vi "Periodic Tasks.vi"() -> ()   [LabVIEW 2019]
doc: "This VI runs in parallel to other tasks. It can contain as many user-defined periodic loops as you need. These can carry out PID or other sorts of timed response."
uses:
  <vilib>/Rock Robotics/WPI/DriverStation/WPI_DriverStationRobotMode2.ctl
  <vilib>/Rock Robotics/WPI/Solenoid/WPI_SolenoidValue.ctl
  <vilib>/Rock Robotics/WPI/Utilities/WPI_GetSetVariantRefNum.vi
  Robot Global Data.vi
  <vilib>/Rock Robotics/WPI/Solenoid/WPI_SolenoidSetEnum.vi
  <vilib>/Rock Robotics/Network Tables/NT Read Number.vi
  <vilib>/Rock Robotics/WPI/ThirdParty/Phoenix-LabVIEW/Motor Controller/Controls/CTRE_Phoenix_MotorControl_ControlMode.ctl
  <vilib>/Rock Robotics/WPI/ThirdParty/REV Robotics/SPARK MAX/Typedef/Spark MAX Control Type.ctl
  <vilib>/Rock Robotics/WPI/ThirdParty/Phoenix-LabVIEW/Motor Controller/Get/CTRE_Phoenix_MotorController_GetQuadratureData.vi
  <vilib>/Rock Robotics/WPI/ThirdParty/Phoenix-LabVIEW/Motor Controller/Get/CTRE_Phoenix_MotorController_GetSelectedSensorData.vi
  <vilib>/Rock Robotics/WPI/ThirdParty/Phoenix-LabVIEW/Motor Controller/Get/CTRE_Phoenix_MotorController_GetVoltage.vi
panel:
  out "Yaw":dbl
  out "status":dbl
  out "X position":dbl
  out "Y position":dbl
  in  "speed":dbl=1000.0
  in  "I Zone":dbl step=0.01
  in  "F Gain":dbl=2.1 step=0.01
  in  "D Gain":dbl=0.005 step=0.01
  in  "I Gain":dbl=0.019999999999999997 step=0.01
  in  "P Gain":dbl=4.0 min=0.0 step=0.01
  out "PID Chart":T1(graph)
  # "Click here to set max"
  # "Click here to set min"
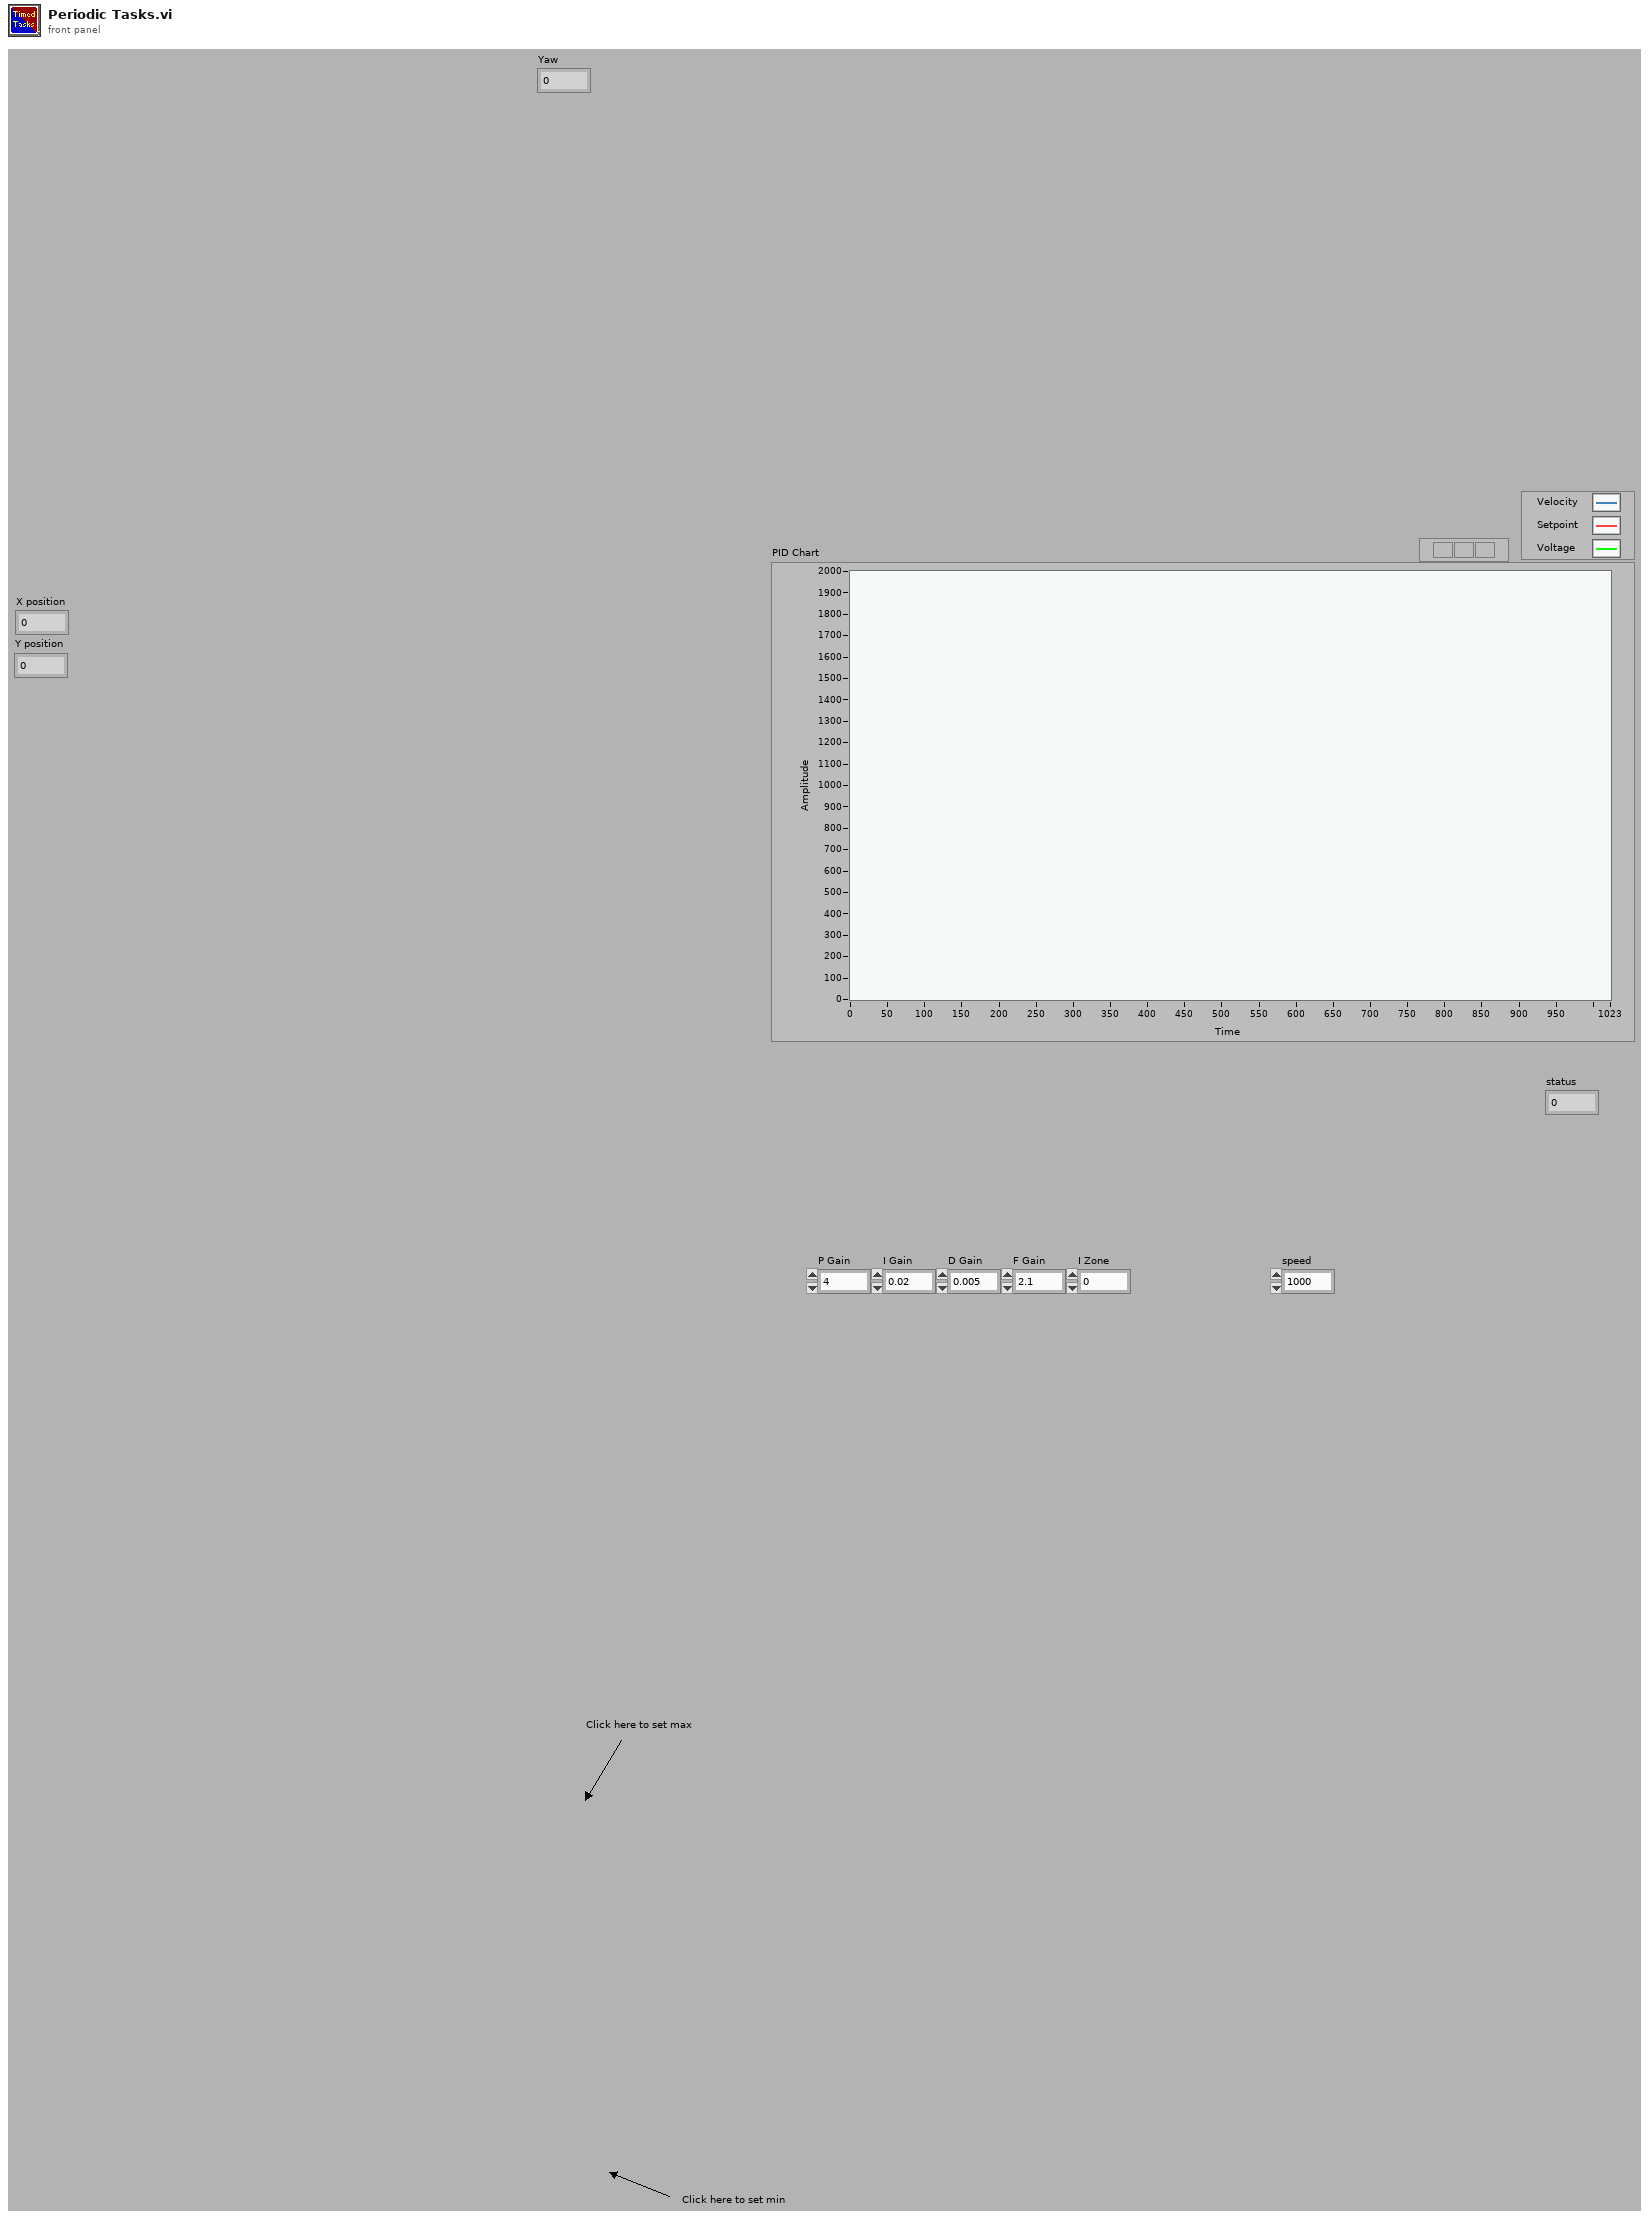
[diagram p1: front panel]
types:
  T1 = cluster{"Sensor Velocity":dbl, "Shooter Top":dbl, "Sensor Velocity":dbl, "Shooter Lower":dbl}
  T2 = typedef "WPI_RobotDriveDevRef.ctl" = cluster{"DevStatus":errorcluster, "Motors[]":T3[], "Square Inputs":bool, "Max Output":dbl}
  T3 = typedef "WPI_MotorControlDeviceRef.ctl" = cluster{"DeviceStatus":errorcluster, "Type":T4, "PWM":cluster{"PWM Channel":T5, "DeadBand":T6}, "CAN":cluster{"Device Number":u8, "SetOutput VI Ref":variant, "GetOutput VI Ref":variant, "Enable VI Ref":variant, "Disable VI Ref":variant, "Data":variant}, "Invert":bool, "DIO PWM":cluster{"PWM \"Enable\" Channel":T5, "DIOChannel":T7, "PWM Rate":dbl}}
  T4 = typedef "WPI_MotorControlType.ctl" = enum16{"PWM", "CAN", "DIO PWM"}
  T5 = typedef "FPGA_DIOPWMChannel.ctl" = enum8{"PWM 0", "PWM 1", "PWM 2", "PWM 3", "PWM 4", "PWM 5", "PWM 6", "PWM 7", "PWM 8", "PWM 9", "PWM MXP 0", "PWM MXP 1", "PWM MXP 2", "PWM MXP 3", "PWM MXP 4", "PWM MXP 5", "PWM MXP 6", "PWM MXP 7", "PWM MXP 8", "PWM MXP 9", "Invalid"}
  T6 = typedef "WPI_PWMDeadband.ctl" = cluster{"Name":string, "maxPositivePwm":i32, "minPositivePwm":i32, "centerPwm":i32, "maxNegativePwm":i32, "minNegativePwm":i32, "angularRange":u16}
  T7 = typedef "FPGA_DIOChannel.ctl" = enum8{"DIO 0", "DIO 1", "DIO 2", "DIO 3", "DIO 4", "DIO 5", "DIO 6", "DIO 7", "DIO 8", "DIO 9", "DIO MXP 0", "DIO MXP 1", "DIO MXP 2", "DIO MXP 3", "DIO MXP 4", "DIO MXP 5", "DIO MXP 6", "DIO MXP 7", "DIO MXP 8", "DIO MXP 9", "DIO MXP 10", "DIO MXP 11", "DIO MXP 12", "DIO MXP 13", "DIO MXP 14", "DIO MXP 15", "SPI Port CS1", "SPI Port CS2", "SPI Port CS3", "SPI Port MISO", "SPI Port MOSI", "Invalid"}
  T8 = typedef "WPI_JoystickDevRef.ctl" = cluster{"Device":T9}
  T9 = typedef "WPI_JoystickDeviceEnum.ctl" = enum16{"USB 0", "USB 1", "USB 2", "USB 3", "USB 4", "USB 5"}
  T10 = typedef "Spark MAX Control Type.ctl" = enum16{"Percent VBus", "Voltage", "Velocity", "Position", "Smart Motion", "Current", "Smart Velocity"}
  T11 = cluster{"[0]":dbl, "[1]":dbl, "[2]":dbl, "[3]":dbl, "[4]":dbl, "[5]":dbl, "[6]":dbl, "[7]":dbl, "[8]":dbl}
  T12 = typedef "CTRE_Phoenix_MotorControl_ControlMode.ctl" = u16
  T13 = cluster{"[0]":bool, "[1]":bool, "[2]":bool, "[3]":bool, "[4]":bool, "[5]":bool, "[6]":bool, "[7]":bool, "[8]":bool}
  T14 = cluster{"JoystickDevRef":T8, "RobotDriveDevRef":T2}
  T15 = typedef "WPI_DriverStationRobotMode2.ctl" = enum16{"Autonomous Disabled", "Autonomous Enabled", "Teleop Disabled", "Teleop Enabled", "Disconnected", "Finish", "Test Disabled", "Test Enabled", "Emergency Stopped"}
  T16 = typedef "WPI_SolenoidValue.ctl" = enum16{"Off", "On", "Forward", "Reverse"}
  T17 = typedef "WPI_SolenoidDevRef.ctl" = cluster{"DevStatus":errorcluster, "Pneumatics Control Module":u8, "Forward Solenoid Channel":T18, "Reverse Solenoid Channel":T18}
  T18 = typedef "WPI_SolenoidChannel.ctl" = enum8{"Solenoid 0", "Solenoid 1", "Solenoid 2", "Solenoid 3", "Solenoid 4", "Solenoid 5", "Solenoid 6", "Solenoid 7", "Invalid"}
  T19 = cluster{"Yaw":dbl, "Roll":dbl, "Pitch":dbl, "Heading":dbl, "Fused Heading":dbl}
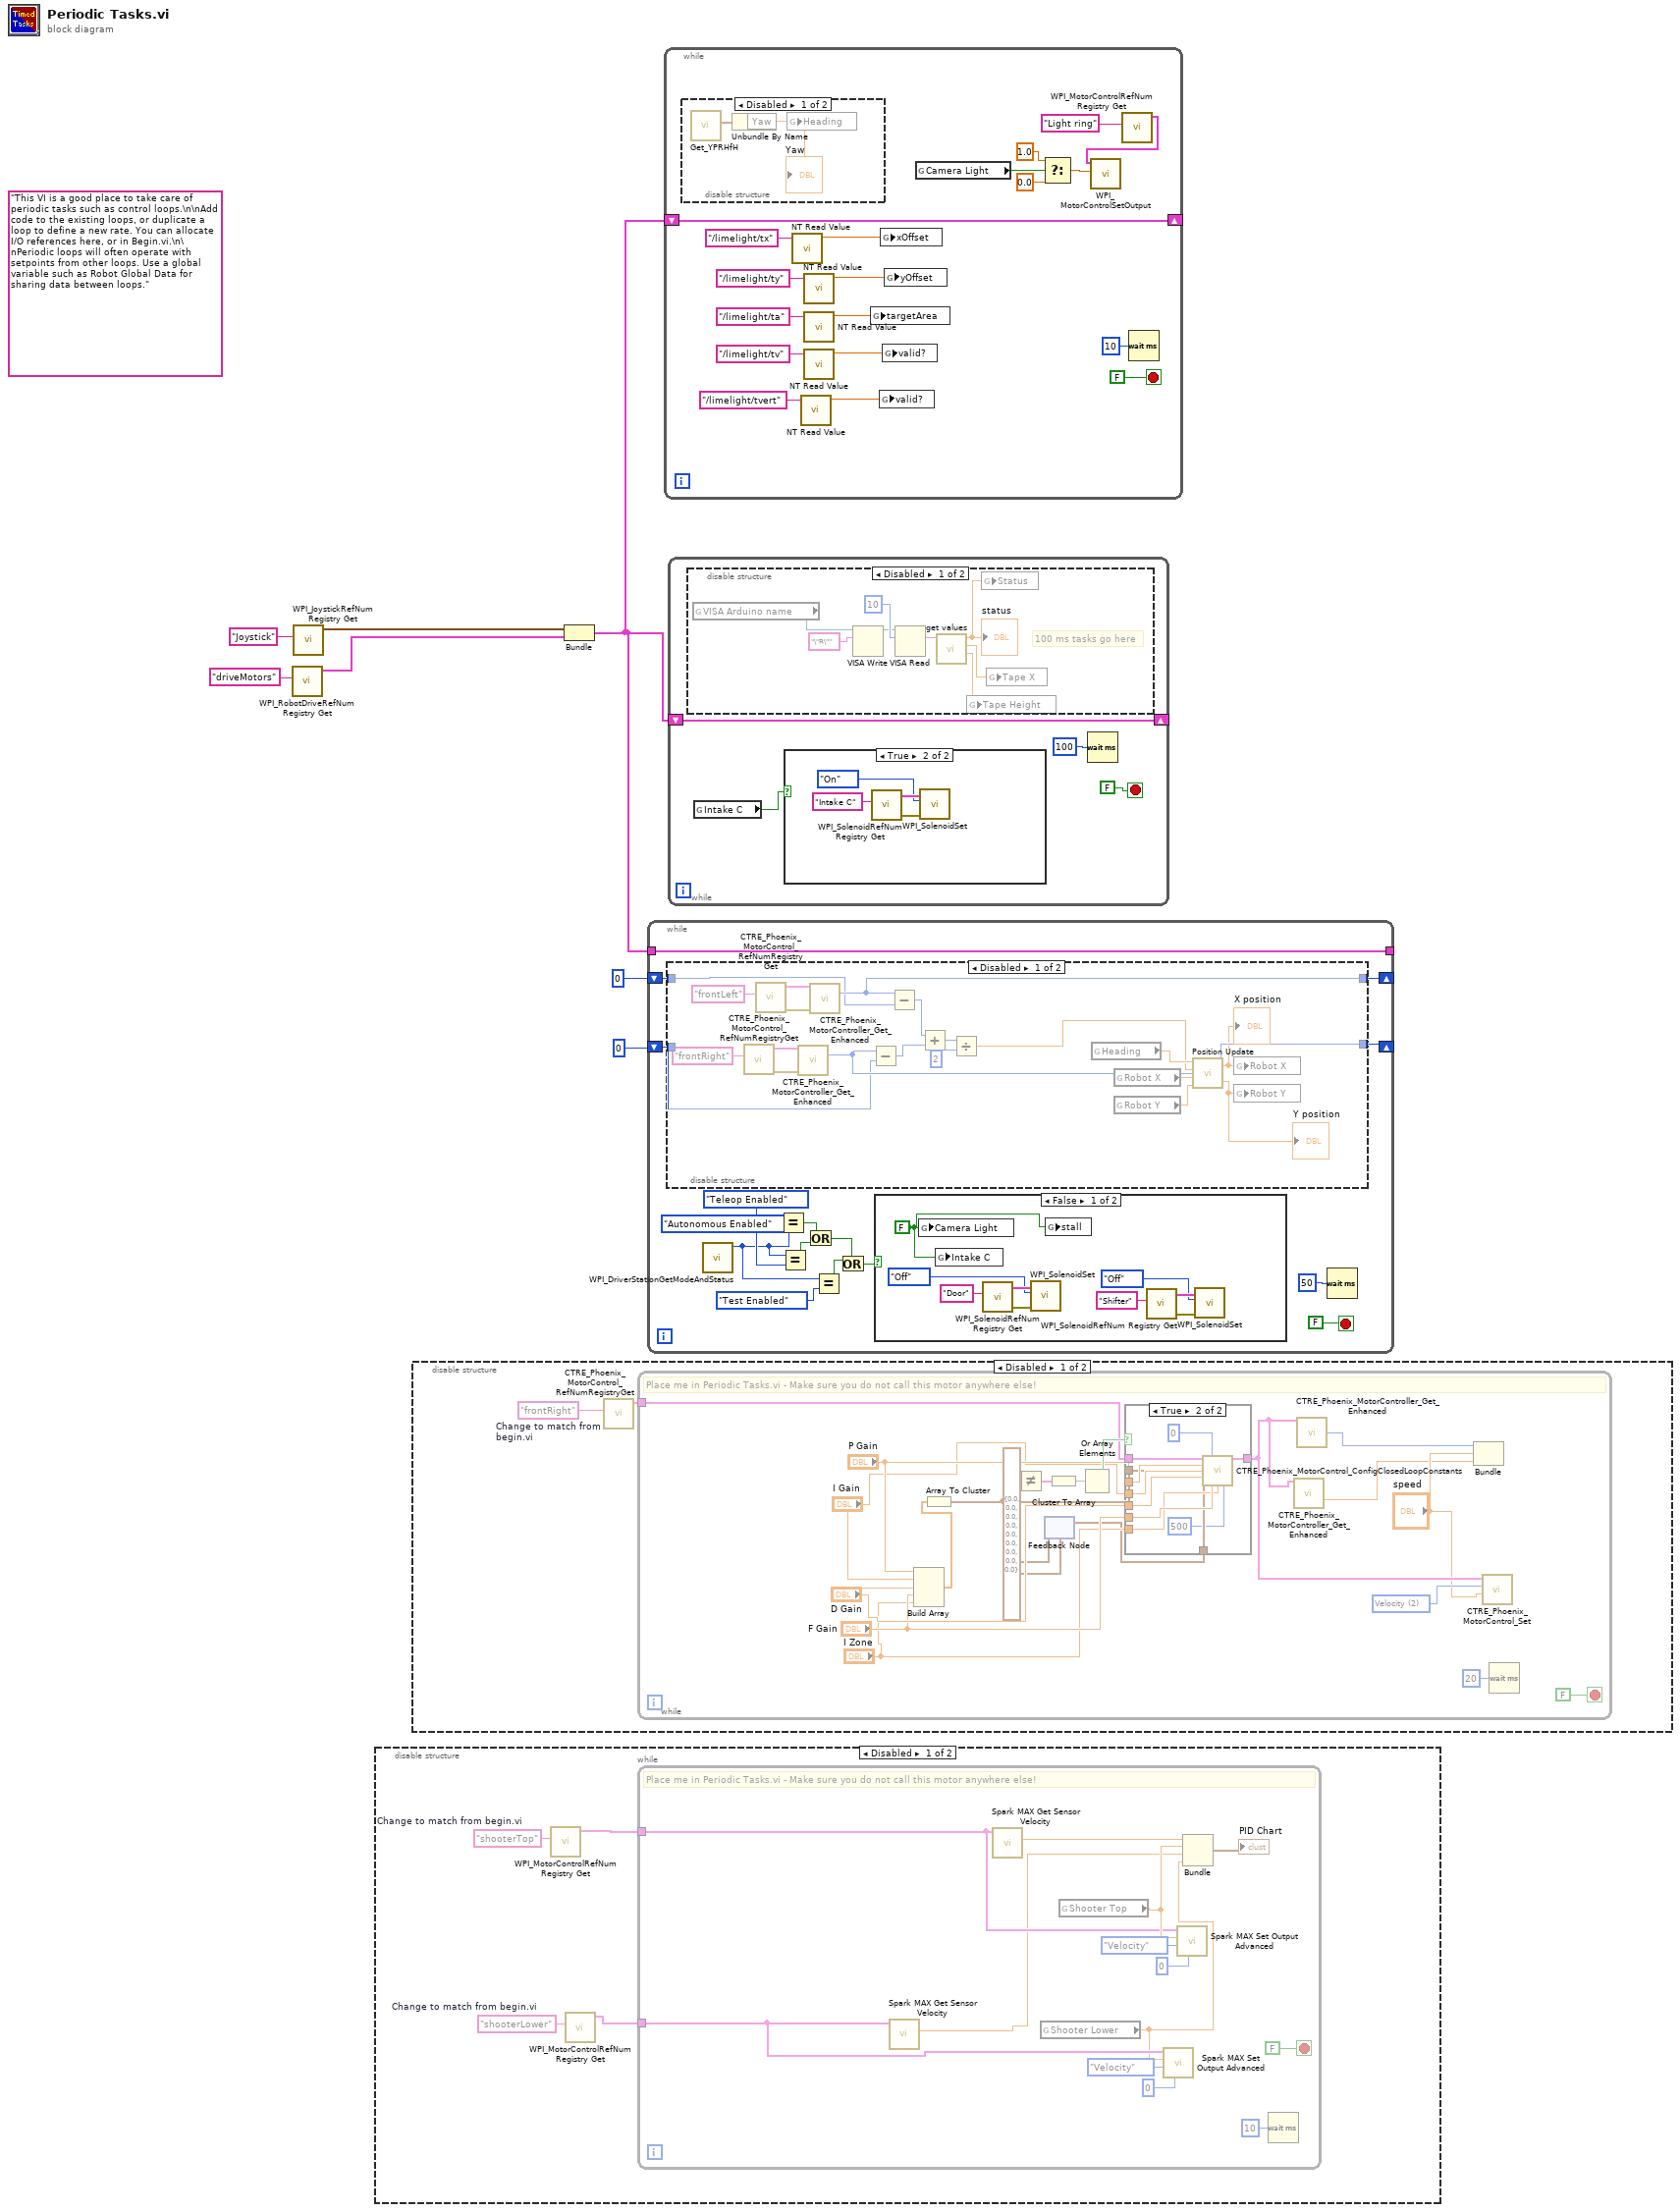
[diagram p0: block diagram]
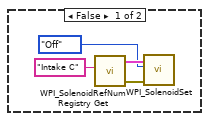
[diagram p4: hidden frame]
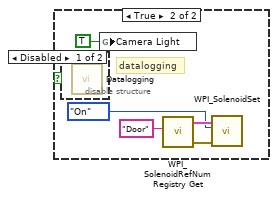
[diagram p6: hidden frame]
diagram:
  (unwired) "This VI is a good place to take care of periodic tasks such as control loops.\n\nAdd code to the existing loops, or duplicate a loop to define a new rate. You can allocate I/O references here, or in Begin.vi.\n\nPeriodic loops will often operate with setpoints from other loops. Use a global variable such as Robot Global Data for sharing data between loops."
  n1 = call <vilib>:"WPI_RobotDriveRefNum Registry Get.vi"("refnum name"="driveMotors") -> ("RobotDriveDevRef"=w4:T2)  [unwired: 1 in, 9 out]
  n2 = call <vilib>:"WPI_JoystickRefNum Registry Get.vi"("refnum name"="Joystick") -> ("JoystickDevRef"=w5:T8)  [unwired: 1 in, 9 out]
  n3 = disable-structure shown="Disabled" {
    frame Disabled {
      w9 = "shooterLower"  # Change to match from begin.vi
      w10 = "shooterTop"  # Change to match from begin.vi
      n4 = call <vilib>:"WPI_MotorControlRefNum Registry Get.vi"("refnum name"=w10) -> ("MotorControlDevRef"=w11:T3)  [unwired: 9 in, 1 out]
      n5 = call <vilib>:"WPI_MotorControlRefNum Registry Get.vi"("refnum name"=w9) -> ("MotorControlDevRef"=w8:T3)  [unwired: 9 in, 1 out]
      n6 = while {
        tunnel: w11 -> [w17]
        tunnel: w8 -> [w14]
        stop <- FALSE stop-if-true
        # "Place me in Periodic Tasks.vi - Make sure you do not call this motor anywhere else!"
        n7 = call <vilib>:"Spark MAX Get Sensor Velocity.vi"("MotorControlDevRef in"=w14) -> ("Sensor Velocity"=w13:dbl)  [unwired: 7 in, 3 out]
        n8 = call <vilib>:"Spark MAX Get Sensor Velocity.vi"("MotorControlDevRef in"=w17) -> ("Sensor Velocity"=w22:dbl)  [unwired: 7 in, 3 out]
        n9 = global read "Robot Global Data.vi" "Shooter Lower"() -> (w12:dbl)
        n10 = global read "Robot Global Data.vi" "Shooter Top"() -> (w18:dbl)
        n11 = call <vilib>:"Spark MAX Set Output Advanced.vi"("PIDF Slot (0)"=0, "Control Mode"=Spark_MAX_Control_Type."Velocity", "Setpoint"=w12, "MotorControlDevRef"=w14) -> ()  [unwired: 6 in, 2 out]
        n12 = call <vilib>:"Spark MAX Set Output Advanced.vi"("PIDF Slot (0)"=0, "Control Mode"=Spark_MAX_Control_Type."Velocity", "Setpoint"=w18, "MotorControlDevRef"=w17) -> ()  [unwired: 6 in, 2 out]
        n13 = Bundle("Sensor Velocity"=w22, "Shooter Top"=w18, "Sensor Velocity"=w13, "Shooter Lower"=w12) -> (→"PID Chart":T1)  [unwired: 1 in]
        n14 = Wait (ms)(milliseconds to wait=u32 10) -> ()  [unwired: 1 out]
      }
    }
    frame Enabled {
    }
  }
  n15 = disable-structure shown="Disabled" {
    frame Disabled {
      w26 = "frontRight"  # Change to match from begin.vi
      n16 = call <vilib>:"CTRE_Phoenix_MotorControl_RefNumRegistryGet.vi"("refnum name"=w26) -> ("PhoenixMotorControlDevRef"=w25:T3)  [unwired: 9 in, 1 out]
      n17 = while {
        tunnel: w25 -> [w27]
        stop <- FALSE stop-if-true
        w43 = T12 2 items=["PercentOutput"=0, "Position"=1, "Velocity"=2, "Current"=3, "Follower"=5, "MotionProfile"=6, "MotionMagic"=7, "MotionProfileArc"=10, "Disabled"=15] ("Control Mode")
        # "Place me in Periodic Tasks.vi - Make sure you do not call this motor anywhere else!"
        n18 = Build Array("P Gain", "I Gain", "D Gain", "F Gain", "I Zone") -> (w41:dbl[])
        n19 = Array To Cluster(array=w41) -> (cluster=w42:T11)
        n20 = feedback #1(T11 {"[0]"=0.0, "[1]"=0.0, "[2]"=0.0, "[3]"=0.0, "[4]"=0.0, "[5]"=0.0, "[6]"=0.0, "[7]"=0.0, "[8]"=0.0}) -> (w33:T11)
        n21 = Not Equal?(x=w42, y=w33) -> (x != y?=w35:T13)
        n22 = Cluster To Array(cluster=w35) -> (array=w46:bool[])
        n23 = Or Array Elements(Boolean array=w46) -> (logical OR=w47:bool)
        n24 = case shown="True" w47 {
          tunnel: w27 -> [w49 w59]
          tunnel: w42 -> [w48 w51]
          tunnel: [w49 w58] -> w32
          tunnel: "P Gain" -> [_ w57]
          tunnel: "I Gain" -> [_ w56]
          tunnel: "D Gain" -> [_ w55]
          tunnel: "F Gain" -> [_ w54]
          tunnel: "I Zone" -> [_ w53]
          tunnel: [w48 w51] -> w34
          frame False {
          }
          frame True {
            n25 = call <vilib>:"CTRE_Phoenix_MotorControl_ConfigClosedLoopConstants.vi"("PhoenixMotorControlDevRef"=w59, "slotIdx"=0, "P"=w57, "I"=w56, "D"=w55, "F"=w54, "I Zone"=w53, "timeoutMs"=500) -> ("PhoenixMotorControlDevRef"=w58:T3)  [unwired: 6 in, 1 out]
          }
        }
        n26 = feedback-in #1(w34) -> ()
        n27 = call-poly <vilib>:"CTRE_Phoenix_MotorController_Get_Enhanced.vi"("PhoenixMotorControlDevRef"=w32) -> ("Bus Voltage"=w28:dbl)  [unwired: 10 in, 4 out]
        n28 = call-poly <vilib>:"CTRE_Phoenix_MotorController_Get_Enhanced.vi"("PhoenixMotorControlDevRef"=w32) -> ("Velocity (Raw Sensor Units per 100 ms)"=w30:i32)  [unwired: 11 in, 3 out]
        n29 = Bundle("Velocity (Raw Sensor Units per 100 ms)"=w30, "speed"="speed", "Bus Voltage"=w28) -> ()  [unwired: 1 in, 1 out]
        n30 = call <vilib>:"CTRE_Phoenix_MotorControl_Set.vi"("Output"="speed", "Control Mode"=w43, "PhoenixMotorControlDevRef"=w32) -> ()  [unwired: 7 in, 2 out]
        n31 = Wait (ms)(milliseconds to wait=u32 20) -> ()  [unwired: 1 out]
      }
    }
    frame Enabled {
    }
  }
  n32 = Bundle("JoystickDevRef"=w5, "RobotDriveDevRef"=w4) -> (w1:T14)  [unwired: 1 out]
  n33 = while {
    tunnel: w1 -> [w75]
    tunnel: [w75] -> _
    shift-right: [w72] -> _
    shift-left: 0 -> [w71]
    shift-right: [w70] -> _
    shift-left: 0 -> [w69]
    stop <- FALSE stop-if-true
    n34 = disable-structure shown="Disabled" {
      disable-tunnel: [w82 _] -> w72
      disable-tunnel: w71 -> [w81 _]
      disable-tunnel: [w80 _] -> w70
      disable-tunnel: w69 -> [w79 _]
      frame Disabled {
        n35 = call <vilib>:"CTRE_Phoenix_MotorControl_RefNumRegistryGet.vi"("refnum name"="frontRight") -> ("error out"=w90:errorcluster, "PhoenixMotorControlDevRef"=w88:T3)  [unwired: 9 in]
        n36 = call <vilib>:"CTRE_Phoenix_MotorControl_RefNumRegistryGet.vi"("refnum name"="frontLeft") -> ("error out"=w92:errorcluster, "PhoenixMotorControlDevRef"=w93:T3)  [unwired: 9 in]
        n37 = call-poly <vilib>:"CTRE_Phoenix_MotorController_Get_Enhanced.vi"("PhoenixMotorControlDevRef"=w88, "error in"=w90) -> ("Quadrature Position"=w80:i32)  [unwired: 10 in, 3 out]
        n38 = call-poly <vilib>:"CTRE_Phoenix_MotorController_Get_Enhanced.vi"("PhoenixMotorControlDevRef"=w93, "error in"=w92) -> ("Quadrature Position"=w82:i32)  [unwired: 10 in, 3 out]
        n39 = Subtract(x=w80, y=w79) -> (x-y=w84:i32)
        n40 = Subtract(x=w82, y=w81) -> (x-y=w83:i32)
        n41 = Add(x=w83, y=w84) -> (x+y=w87:i32)
        n42 = Divide(x=w87, y=2) -> (x/y=w76:dbl)
        n43 = global read "Robot Global Data.vi" "Heading"() -> (w85:dbl)
        n44 = global read "Robot Global Data.vi" "Robot X"() -> (w94:dbl)
        n45 = global read "Robot Global Data.vi" "Robot Y"() -> (w95:dbl)
        n46 = call "Position Update.vi"("Y position in"=w95, "X position in"=w94, "Distance"=w76, "Heading"=w85) -> ("Y position"=w77:dbl, "X position"=w78:dbl)
        "X position" <- w78
        "Y position" <- w77
        n47 = global write "Robot Global Data.vi" "Robot X"(w78) -> ()
        n48 = global write "Robot Global Data.vi" "Robot Y"(w77) -> ()
      }
      frame Enabled {
      }
    }
    n49 = call <vilib>:"WPI_DriverStationGetModeAndStatus.vi"() -> ("Robot Mode"=w65:T15)  [unwired: 10 in, 1 out]
    n50 = Equal?(x=WPI_DriverStationRobotMode2."Autonomous Enabled" ("Robot Mode"), y=w65) -> (x = y?=w68:bool)
    n51 = Equal?(x=w65, y=WPI_DriverStationRobotMode2."Teleop Enabled" ("Robot Mode")) -> (x = y?=w62:bool)
    n52 = Or(x=w68, y=w62) -> (x .or. y?=w61:bool)
    n53 = Equal?(x=w65, y=WPI_DriverStationRobotMode2."Test Enabled" ("Robot Mode")) -> (x = y?=w66:bool)
    n54 = Or(x=w66, y=w61) -> (x .or. y?=w63:bool)
    n55 = case shown="False" w63 {
      frame False {
        w96 = FALSE ("Camera Light")
        n56 = global write "Robot Global Data.vi" "Camera Light"(w96) -> ()
        n57 = global write "Robot Global Data.vi" "Intake C"(w96) -> ()
        n58 = call <vilib>:"WPI_SolenoidRefNum Registry Get.vi"("refnum name"="Door") -> ("error out"=w104:errorcluster, "SolenoidDevRef"=w103:T17)  [unwired: 9 in]
        n59 = call-poly <vilib>:"WPI_SolenoidSet.vi"("error in (no error)"=w104, "Value"=WPI_SolenoidValue."Off", "SolenoidDevRef"=w103) -> ()  [unwired: 7 in, 2 out]
        n60 = global write "Robot Global Data.vi" "stall"(w96) -> ()
        n61 = call <vilib>:"WPI_SolenoidRefNum Registry Get.vi"("refnum name"="Shifter") -> ("error out"=w100:errorcluster, "SolenoidDevRef"=w99:T17)  [unwired: 9 in]
        n62 = call-poly <vilib>:"WPI_SolenoidSet.vi"("error in (no error)"=w100, "Value"=WPI_SolenoidValue."Off", "SolenoidDevRef"=w99) -> ()  [unwired: 7 in, 2 out]
      }
      frame True {
        # "datalogging"
        n63 = disable-structure shown="Disabled" {
          frame Disabled {
            n64 = call "Datalogging.vi"() -> ()  [unwired: 12 in]
          }
          frame Enabled {
          }
        }
        n65 = global write "Robot Global Data.vi" "Camera Light"(TRUE ("Camera Light")) -> ()
        n66 = call <vilib>:"WPI_SolenoidRefNum Registry Get.vi"("refnum name"="Door") -> ("error out"=w108:errorcluster, "SolenoidDevRef"=w107:T17)  [unwired: 9 in]
        n67 = call-poly <vilib>:"WPI_SolenoidSet.vi"("error in (no error)"=w108, "Value"=WPI_SolenoidValue."On", "SolenoidDevRef"=w107) -> ()  [unwired: 7 in, 2 out]
      }
    }
    n68 = Wait (ms)(milliseconds to wait=u32 50) -> ()  [unwired: 1 out]
  }
  n69 = while {
    shift-right: [w126] -> _
    shift-left: w1 -> [w126]
    stop <- FALSE stop-if-true
    n70 = disable-structure shown="Disabled" {
      frame Disabled {
        n71 = call <vilib>:"Get_YPRHfH.vi"() -> ("YRPHfH"=w130:T19)  [unwired: 11 in]
        n72 = Unbundle By Name(w130) -> ("Yaw"=w129:dbl)
        "Yaw" <- w129
        n73 = global write "Robot Global Data.vi" "Heading"(w129) -> ()
      }
      frame Enabled {
      }
    }
    n74 = call-poly <vilib>:"NT Read Value.vi"("Name"="/limelight/tx") -> ("Numeric"=w121:dbl)  [unwired: 9 in, 1 out]
    n75 = call-poly <vilib>:"NT Read Value.vi"("Name"="/limelight/tvert") -> ("Numeric"=w116:dbl)  [unwired: 9 in, 1 out]
    n76 = call-poly <vilib>:"NT Read Value.vi"("Name"="/limelight/ty") -> ("Numeric"=w120:dbl)  [unwired: 9 in, 1 out]
    n77 = call-poly <vilib>:"NT Read Value.vi"("Name"="/limelight/ta") -> ("Numeric"=w119:dbl)  [unwired: 9 in, 1 out]
    n78 = call-poly <vilib>:"NT Read Value.vi"("Name"="/limelight/tv") -> ("Numeric"=w118:dbl)  [unwired: 9 in, 1 out]
    n79 = global write "Robot Global Data.vi" "targetArea"(w119) -> ()
    n80 = global write "Robot Global Data.vi" "valid?"(w116) -> ()
    n81 = global write "Robot Global Data.vi" "xOffset"(w121) -> ()
    n82 = global write "Robot Global Data.vi" "valid?"(w118) -> ()
    n83 = global write "Robot Global Data.vi" "yOffset"(w120) -> ()
    n84 = global read "Robot Global Data.vi" "Camera Light"() -> (w113:bool)
    n85 = Select(t=1.0, s=w113, f=0.0) -> (s? t:f=w114:dbl)
    n86 = call <vilib>:"WPI_MotorControlRefNum Registry Get.vi"("refnum name"="Light ring") -> ("MotorControlDevRef"=w110:T3)  [unwired: 9 in, 1 out]
    n87 = call <vilib>:"WPI_MotorControlSetOutput.vi"("Output"=w114, "MotorControlDevRef"=w110) -> ()  [unwired: 7 in, 3 out]
    n88 = Wait (ms)(milliseconds to wait=u32 10) -> ()  [unwired: 1 out]
  }
  n89 = while {
    shift-right: [w132] -> _
    shift-left: w1 -> [w132]
    stop <- FALSE stop-if-true
    n90 = disable-structure shown="Disabled" {
      frame Disabled {
        # "100 ms tasks go here"
        n91 = global read "Robot Global Data.vi" "VISA Arduino name"() -> (w137:refnum<visa-resource-name>)
        n92 = VISA Write(VISA resource name=w137, write buffer="\"R\"") -> (VISA resource name out=w136:refnum<visa-resource-name>)  [unwired: 1 in, 2 out]
        n93 = VISA Read(VISA resource name=w136, byte count=u32 10) -> (read buffer=w139:string)  [unwired: 1 in, 3 out]
        n94 = call "get values.vi"("USB In"=w139) -> ("insidex (0-319)"=w140:dbl, "averagex (0-319)"=w141:dbl, "status"=w142:dbl)  [unwired: 8 in]
        "status" <- w142
        n95 = global write "Robot Global Data.vi" "Tape Height"(w140) -> ()
        n96 = global write "Robot Global Data.vi" "Status"(w142) -> ()
        n97 = global write "Robot Global Data.vi" "Tape X"(w141) -> ()
      }
      frame Enabled {
      }
    }
    n98 = global read "Robot Global Data.vi" "Intake C"() -> (w131:bool)
    n99 = case shown="True" w131 {
      frame False {
        n100 = call <vilib>:"WPI_SolenoidRefNum Registry Get.vi"("refnum name"="Intake C") -> ("error out"=w146:errorcluster, "SolenoidDevRef"=w145:T17)  [unwired: 9 in]
        n101 = call-poly <vilib>:"WPI_SolenoidSet.vi"("error in (no error)"=w146, "Value"=WPI_SolenoidValue."Off", "SolenoidDevRef"=w145) -> ()  [unwired: 7 in, 2 out]
      }
      frame True {
        n102 = call <vilib>:"WPI_SolenoidRefNum Registry Get.vi"("refnum name"="Intake C") -> ("error out"=w150:errorcluster, "SolenoidDevRef"=w149:T17)  [unwired: 9 in]
        n103 = call-poly <vilib>:"WPI_SolenoidSet.vi"("error in (no error)"=w150, "Value"=WPI_SolenoidValue."On", "SolenoidDevRef"=w149) -> ()  [unwired: 7 in, 2 out]
      }
    }
    n104 = Wait (ms)(milliseconds to wait=u32 100) -> ()  [unwired: 1 out]
  }
